vi "Pre-Install Custom Action.vi"(10 "Variant":variant) -> (0 "error out":errorcluster)   [LabVIEW 2026]
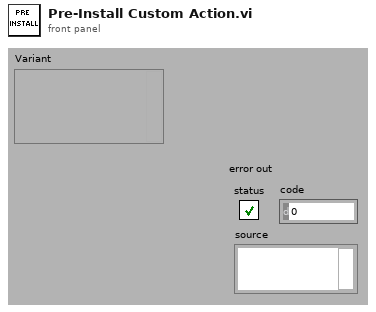
[diagram p1: front panel]
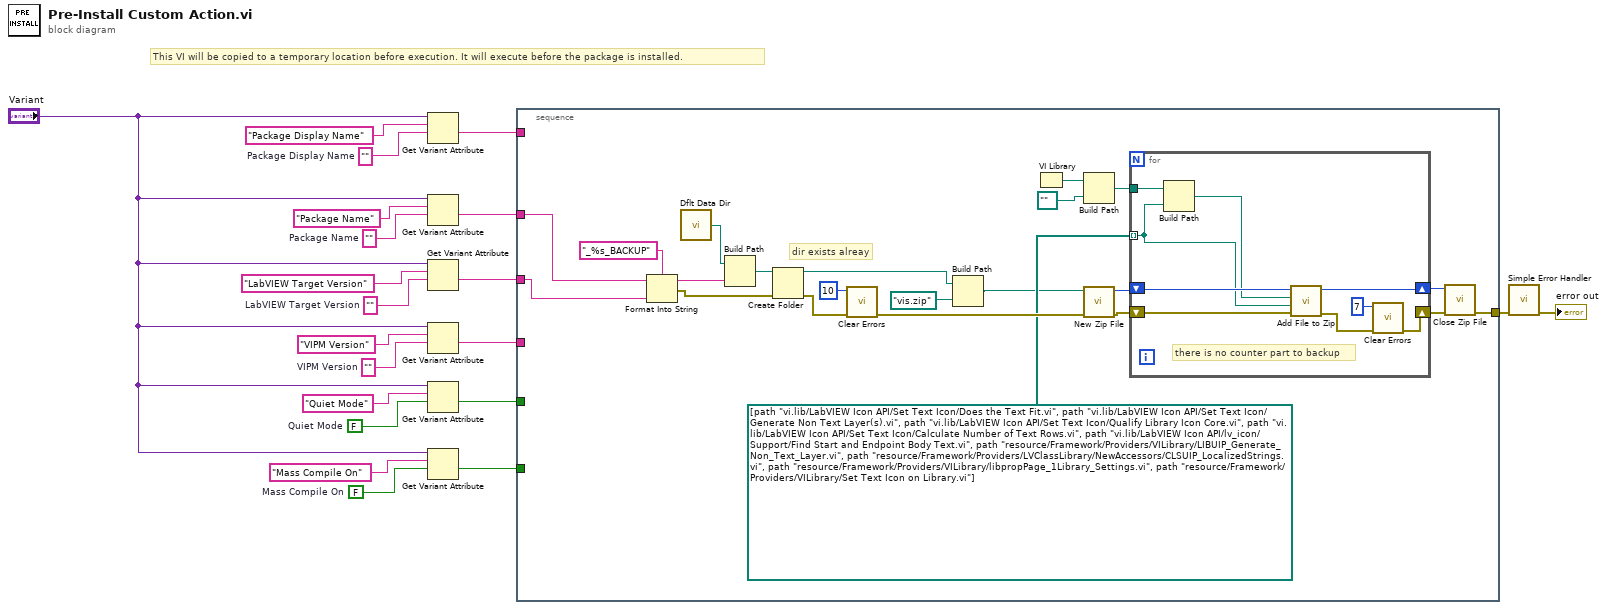
[diagram p0: block diagram]
diagram:
  w3 = FALSE  # Mass Compile On
  w5 = ""  # Package Display Name
  w12 = FALSE  # Quiet Mode
  w15 = ""  # VIPM Version
  w17 = ""  # LabVIEW Target Version
  w19 = ""  # Package Name
  # "This VI will be copied to a temporary location before execution. It will execute before the package is installed."
  n1 = Get Variant Attribute(Variant="Variant", name="Package Display Name", default value (empty Variant)=w5) -> (value=w11:string)  [unwired: 1 in, 3 out]
  n2 = Get Variant Attribute(Variant="Variant", name="Package Name", default value (empty Variant)=w19) -> (value=w10:string)  [unwired: 1 in, 3 out]
  n3 = Get Variant Attribute(Variant="Variant", name="LabVIEW Target Version", default value (empty Variant)=w17) -> (value=w9:string)  [unwired: 1 in, 3 out]
  n4 = Get Variant Attribute(Variant="Variant", name="VIPM Version", default value (empty Variant)=w15) -> (value=w8:string)  [unwired: 1 in, 3 out]
  n5 = Get Variant Attribute(Variant="Variant", name="Quiet Mode", default value (empty Variant)=w12) -> (value=w7:bool)  [unwired: 1 in, 3 out]
  n6 = Get Variant Attribute(Variant="Variant", name="Mass Compile On", default value (empty Variant)=w3) -> (value=w6:bool)  [unwired: 1 in, 3 out]
  n7 = stacked-sequence {
    tunnel: w11 -> [_]
    tunnel: w10 -> [w26]
    tunnel: w9 -> [w23]
    tunnel: w8 -> [_]
    tunnel: w7 -> [_]
    tunnel: w6 -> [_]
    tunnel: [w29] -> w2
    frame #0 {
      # "dir exists alreay"
      n8 = Format Into String(format string="_%s_BACKUP", initial string=w26, w23) -> (resulting string=w25:string, error out=w22:errorcluster)  [unwired: 1 in]
      n9 = call <vilib>:"Dflt Data Dir.vi"() -> ("App:Default Data Directory"=w39:path)
      n10 = Build Path(base path=w39, name or relative path=w25) -> (appended path=w31:path)
      n11 = Create Folder(path (use dialog)=w31, error in=w22) -> (created path=w27:path, error out=w37:errorcluster)  [unwired: 1 in, 1 out]
      n12 = call <vilib>:"Clear Errors.vi"("error in (no error)"=w37, "specific error code to clear (0: all)"=10) -> ("error out"=w36:errorcluster)  [unwired: 4 in, 1 out]
      n13 = Build Path(base path=w27, name or relative path=path "vis.zip") -> (appended path=w28:path)
      n14 = VI Library() -> (path=w35:path)
      n15 = Build Path(base path=w35, name or relative path=path "..") -> (appended path=w33:path)
      n16 = call <vilib>:"New Zip File.vi"("error in (no error)"=w36, "target"=w28) -> ("error out"=w42:errorcluster, "zip file out"=w43:i64)  [unwired: 3 in, 1 out]
      n17 = for {
        tunnel: path[] [path "vi.lib/LabVIEW Icon API/Set Text Icon/Does the Text Fit.vi", path "vi.lib/LabVIEW Icon API/Set Text Icon/Generate Non Text Layer(s).vi", path "vi.lib/LabVIEW Icon API/Set Text Icon/Qualify Library Icon Core.vi", path "vi.lib/LabVIEW Icon API/Set Text Icon/Calculate Number of Text Rows.vi", path "vi.lib/LabVIEW Icon API/lv_icon/Support/Find Start and Endpoint Body Text.vi", path "resource/Framework/Providers/VILibrary/LIBUIP_Generate_Non_Text_Layer.vi", path "resource/Framework/Providers/LVClassLibrary/NewAccessors/CLSUIP_LocalizedStrings.vi", path "resource/Framework/Providers/VILibrary/libpropPage_1Library_Settings.vi", path "resource/Framework/Providers/VILibrary/Set Text Icon on Library.vi"] ("packages member source files") -> [w44] mode=indexing
        shift-right: [w47] -> w41
        shift-left: w42 -> [w49]
        shift-right: [w50] -> w40
        shift-left: w43 -> [w51]
        tunnel: w33 -> [w45]
        # "there is no counter part to backup"
        n18 = Build Path(base path=w45, name or relative path=w44) -> (appended path=w48:path)
        n19 = call <vilib>:"Add File to Zip.vi"("error in (no error)"=w49, "destination path in zip"=w44, "source file path"=w48, "zip file in"=w51) -> ("error out"=w52:errorcluster, "zip file out"=w50:i64)  [unwired: 6 in]
        n20 = call <vilib>:"Clear Errors.vi"("error in (no error)"=w52, "specific error code to clear (0: all)"=7) -> ("error out"=w47:errorcluster)  [unwired: 4 in, 1 out]
      }
      n21 = call <vilib>:"Close Zip File.vi"("error in (no error)"=w41, "zip file in"=w40) -> ("error out"=w29:errorcluster)  [unwired: 5 in]
    }
  }
  n22 = call <vilib>:"Simple Error Handler.vi"("error in (no error)"=w2) -> ("error out"=→"error out":errorcluster)  [unwired: 4 in, 4 out]
